vi "Fpga-Get-Integer32.vi"(6 "upper":u16=7, 7 "lower":u16=2, 9 "Reset":bool, 10 "DataIn":u8, 11 "Index":u16) -> (2 "Valid":bool, 3 "UInt32":u32)   [LabVIEW 2016]
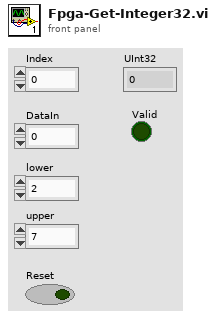
[diagram p1: front panel]
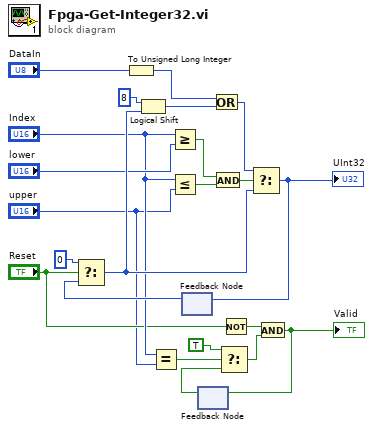
[diagram p0: block diagram]
diagram:
  n1 = To Unsigned Long Integer(number="DataIn") -> (unsigned 32bit integer=w14:u32)
  n2 = Equal?(x="Index", y="upper") -> (x = y?=w8:bool)
  n3 = Greater Or Equal?(x="Index", y="lower") -> (x >= y?=w16:bool)
  n4 = Less Or Equal?(x="Index", y="upper") -> (x <= y?=w17:bool)
  n5 = feedback #1() -> (w20:u32)  [unwired: 1 in]
  n6 = Select(t=u32 0, s="Reset", f=w20) -> (s? t:f=w21:u32)
  n7 = Logical Shift(y=i16 8, x=w21) -> (x << y=w11:u32)
  n8 = feedback #2() -> (w6:bool)  [unwired: 1 in]
  n9 = Or(x=w14, y=w11) -> (x .or. y?=w12:u32)
  n10 = And(x=w16, y=w17) -> (x .and. y?=w15:bool)
  n11 = Select(t=TRUE, s=w8, f=w6) -> (s? t:f=w3:bool)
  n12 = Not(x="Reset") -> (.not. x?=w4:bool)
  n13 = Select(t=w12, s=w15, f=w21) -> (s? t:f=w19:u32)
  "UInt32" <- w19
  n14 = feedback-in #1(w19) -> ()
  n15 = And(x=w4, y=w3) -> (x .and. y?=w2:bool)
  "Valid" <- w2
  n16 = feedback-in #2(w2) -> ()
